vi "se_scaleOffsetRotateOutput.vi"(6 "inputValid":bool, 8 "scanSize":T1, 9 "outputMatrix":T4, 10 "scanOffset":cluster{"x":fxp<+/-,16,1>, "y":fxp<+/-,16,1>}, 11 "input":T3) -> (0 "outputValid":bool, 2 "outputInt":cluster{"x":i16, "y":i16}, 3 "outputNorm":T2)   [LabVIEW 2016]
uses:
  <vilib>/rvi/FXPMathLib/FxpMul/XNode/nifxpmath_Multiplier.xnode
  <vilib>/rvi/FXPMathLib/FxpAdd/XNode/nifxpmath_Add.xnode
  <vilib>/rvi/FXPMathLib/FxpInterpret/XNode/nifxpmath_Interpret.xnode
  <vilib>/rvi/FXPMathLib/sim/FxpSim.dll
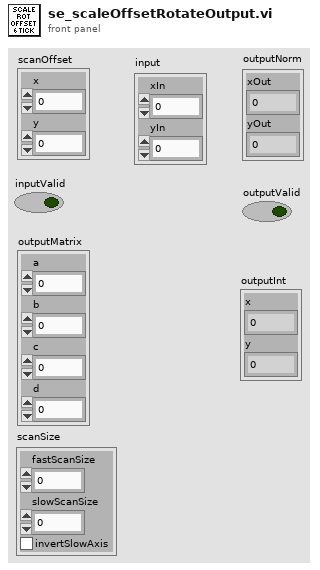
[diagram p1: front panel]
types:
  T1 = cluster{"fastScanSize":fxp<+,17,1>, "slowScanSize":fxp<+,17,1>, "invertSlowAxis":bool}
  T2 = cluster{"xOut":fxp<+/-,18,2>, "yOut":fxp<+/-,18,2>}
  T3 = cluster{"xIn":fxp<+/-,19,2>, "yIn":fxp<+/-,19,2>}
  T4 = cluster{"a":fxp<+/-,18,2>, "b":fxp<+/-,18,2>, "c":fxp<+/-,18,2>, "d":fxp<+/-,18,2>}
  T5 = cluster{"x+y":fxp<+/-,18,2>, "x+y":fxp<+/-,18,2>}
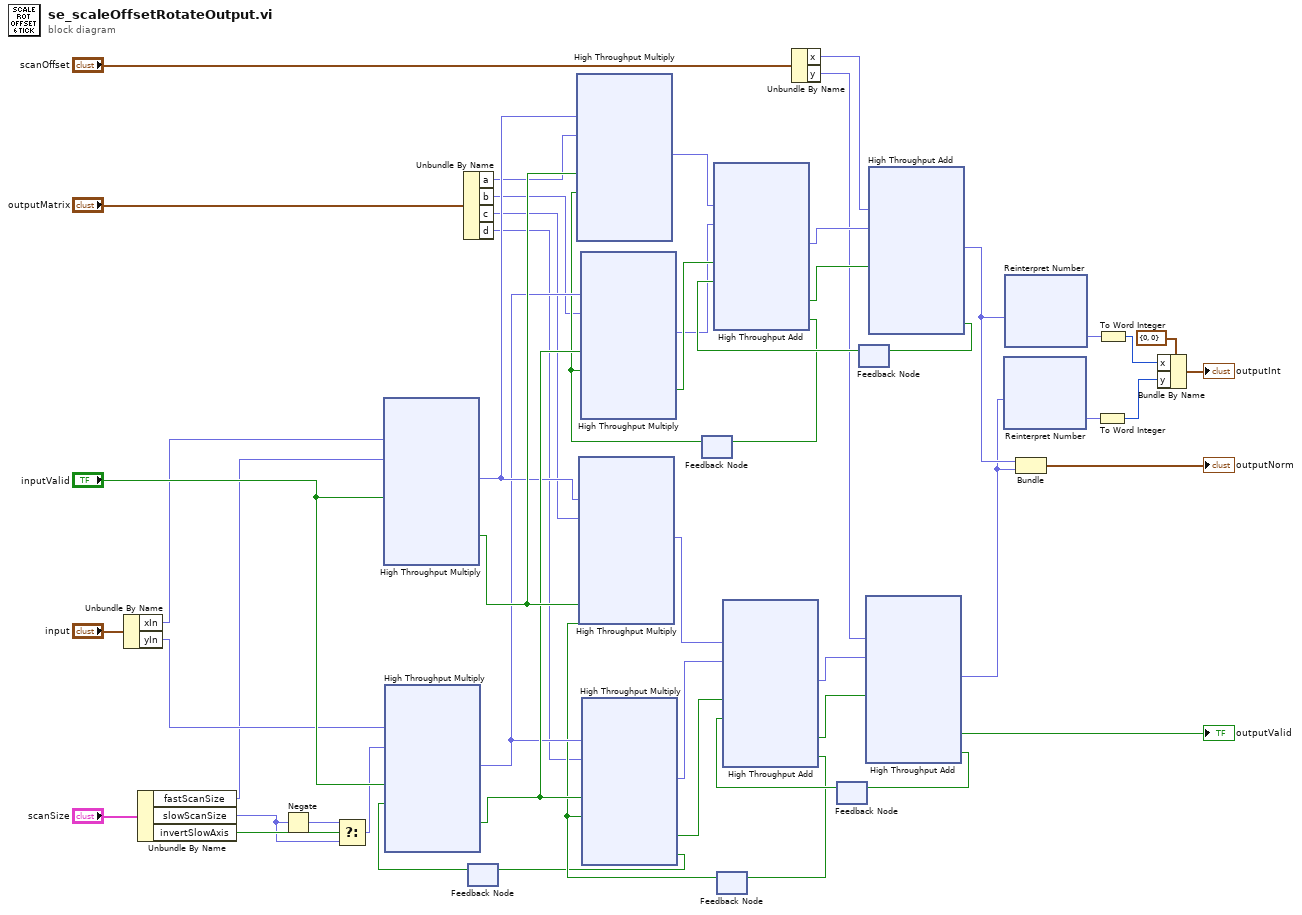
[diagram p0: block diagram]
diagram:
  n1 = Unbundle By Name("input") -> ("xIn"=w17:fxp<+/-,19,2>, "yIn"=w16:fxp<+/-,19,2>)
  n2 = Unbundle By Name("scanSize") -> ("fastScanSize"=w13:fxp<+,17,1>, "slowScanSize"=w2:fxp<+,17,1>, "invertSlowAxis"=w6:bool)
  n3 = Negate(x=w2) -> (-x=w5:fxp<+/-,18,2>)
  n4 = Select(t=w5, s=w6, f=w2) -> (s? t:f=w1:fxp<+/-,18,2>)
  n5 = xnode ("High Throughput Multiply")("x"=w17, "y"=w13, "input valid"="inputValid") -> ("x*y"=w39:fxp<+/-,18,2>, "output valid"=w42:bool)  [unwired: 1 in, 1 out]
  n6 = Unbundle By Name("outputMatrix") -> ("a"=w23:fxp<+/-,18,2>, "b"=w24:fxp<+/-,18,2>, "c"=w25:fxp<+/-,18,2>, "d"=w30:fxp<+/-,18,2>)
  n7 = feedback #1() -> (w40:bool)  [unwired: 1 in]
  n8 = xnode ("High Throughput Multiply")("x"=w16, "y"=w1, "input valid"="inputValid", "ready for output (T)"=w40) -> ("x*y"=w38:fxp<+/-,18,2>, "output valid"=w41:bool)  [unwired: 1 out]
  n9 = feedback #2() -> (w36:bool)  [unwired: 1 in]
  n10 = xnode ("High Throughput Multiply")("x"=w39, "y"=w23, "input valid"=w42, "ready for output (T)"=w36) -> ("x*y"=w26:fxp<+/-,18,2>)  [unwired: 2 out]
  n11 = xnode ("High Throughput Multiply")("x"=w38, "y"=w24, "input valid"=w41, "ready for output (T)"=w36) -> ("x*y"=w27:fxp<+/-,18,2>, "output valid"=w32:bool)  [unwired: 1 out]
  n12 = feedback #3() -> (w37:bool)  [unwired: 1 in]
  n13 = xnode ("High Throughput Multiply")("x"=w39, "y"=w25, "input valid"=w42, "ready for output (T)"=w37) -> ("x*y"=w28:fxp<+/-,18,2>)  [unwired: 2 out]
  n14 = xnode ("High Throughput Multiply")("x"=w38, "y"=w30, "input valid"=w41, "ready for output (T)"=w37) -> ("x*y"=w29:fxp<+/-,18,2>, "output valid"=w33:bool, "ready for input"=w31:bool)
  n15 = feedback-in #1(w31) -> ()
  n16 = Unbundle By Name("scanOffset") -> ("x"=w21:fxp<+/-,16,1>, "y"=w20:fxp<+/-,16,1>)
  n17 = feedback #4() -> (w49:bool)  [unwired: 1 in]
  n18 = xnode ("High Throughput Add")("x"=w28, "y"=w29, "input valid"=w33, "ready for output (T)"=w49) -> ("x+y"=w50:fxp<+/-,18,2>, "output valid"=w44:bool, "ready for input"=w34:bool)
  n19 = feedback-in #3(w34) -> ()
  n20 = feedback #5() -> (w47:bool)  [unwired: 1 in]
  n21 = xnode ("High Throughput Add")("x"=w26, "y"=w27, "input valid"=w32, "ready for output (T)"=w47) -> ("x+y"=w51:fxp<+/-,18,2>, "output valid"=w45:bool, "ready for input"=w35:bool)
  n22 = feedback-in #2(w35) -> ()
  n23 = xnode ("High Throughput Add")("x"=w20, "y"=w50, "input valid"=w44) -> ("x+y"=w3:fxp<+/-,18,2>, "output valid"=→"outputValid":bool, "ready for input"=w48:bool)  [unwired: 1 in]
  n24 = feedback-in #4(w48) -> ()
  n25 = xnode ("High Throughput Add")("x"=w21, "y"=w51, "input valid"=w45) -> ("x+y"=w8:fxp<+/-,18,2>, "ready for input"=w46:bool)  [unwired: 1 in, 1 out]
  n26 = feedback-in #5(w46) -> ()
  n27 = xnode "Reinterpret Number"("x"=w3) -> ("y"=w11:fxp<+/-,18,17>)
  n28 = xnode "Reinterpret Number"("x"=w8) -> ("y"=w12:fxp<+/-,18,17>)
  n29 = Bundle("x+y"=w8, "x+y"=w3) -> (→"outputNorm":T5)  [unwired: 1 in]
  n30 = To Word Integer(number=w11) -> (16bit integer=w4:i16)
  n31 = To Word Integer(number=w12) -> (16bit integer=w9:i16)
  n32 = Bundle By Name(cluster=cluster{"x":i16, "y":i16} {"x"=0, "y"=0} ("Element"), "x"=w9, "y"=w4) -> (→"outputInt":cluster{"x":i16, "y":i16})
